vi "SVFA Concatenate Spectra (XY) (1 Ch).vi"(10 "spectrum (high frequency)":cluster{"X":dbl[], "Y":dbl[]}, 11 "spectrum (low frequency)":cluster{"X":dbl[], "Y":dbl[]}) -> (3 "concatenated spectrum":cluster{"X":dbl[], "Y":dbl[]})   [LabVIEW 2017]
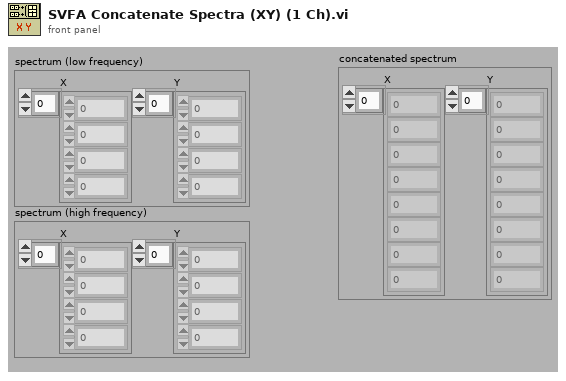
[diagram p1: front panel]
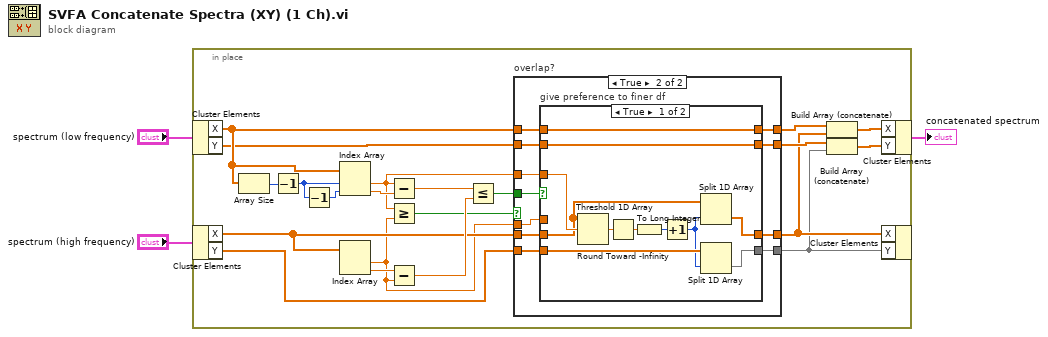
[diagram p0: block diagram]
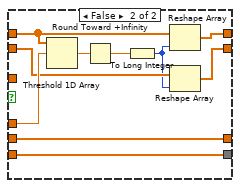
[diagram p3: hidden frame]
diagram:
  n1 = in-place {
    n2 = in-place-cluster #1("spectrum (low frequency)") -> ("X"=w14:dbl[], "Y"=w12:dbl[])
    n3 = in-place-cluster #2("spectrum (high frequency)") -> ("X"=w10:dbl[], "Y"=w7:dbl[])
    n4 = Array Size(array=w14) -> (size(s)=w22:i32)
    n5 = Decrement(x=w22) -> (x-1=w21:i32)
    n6 = Decrement(x=w21) -> (x-1=w20:i32)
    n7 = Index Array(array=w14, index #1=w21, index #2=w20) -> (element #1=w6:dbl, element #2=w18:dbl)
    n8 = Index Array(array=w10) -> (element #1=w5:dbl, element #2=w19:dbl)  [unwired: 2 in]
    n9 = Subtract(x=w6, y=w18) -> (x-y=w17:dbl)
    n10 = Greater Or Equal?(x=w6, y=w5) -> (x >= y?=w4:bool)
    n11 = Subtract(x=w19, y=w5) -> (x-y=w16:dbl)
    n12 = Less Or Equal?(x=w17, y=w16) -> (x <= y?=w15:bool)
    n13 = case "overlap?" shown="True" w4 {
      tunnel: w15 -> [_ w39]
      tunnel: w14 -> [w28 w38]
      tunnel: [w28 w37] -> w13
      tunnel: w12 -> [w27 w36]
      tunnel: [w27 w35] -> w11
      tunnel: w10 -> [w26 w34]
      tunnel: [w26 w33] -> w9
      tunnel: [w25 w32] -> w8
      tunnel: w7 -> [w25 w31]
      tunnel: w6 -> [_ w30]
      tunnel: w5 -> [_ w29]
      frame False {
      }
      frame True {
        n14 = case "give preference to finer df" shown="True" w39 {
          tunnel: w34 -> [w49 w55]
          tunnel: w30 -> [w50 _]
          tunnel: [w48 w55] -> w33
          tunnel: w31 -> [w44 w54]
          tunnel: [w47 w54] -> w32
          tunnel: w29 -> [_ w58]
          tunnel: w38 -> [w46 w57]
          tunnel: [w46 w53] -> w37
          tunnel: w36 -> [w45 w56]
          tunnel: [w45 w52] -> w35
          frame True {
            n15 = Threshold 1D Array(2:w50, 3:w49) -> (0:w43:dbl)  [unwired: 1 in]
            n16 = Round Toward -Infinity(1:w43) -> (0:w42:dbl)
            n17 = To Long Integer(number=w42) -> (32bit integer=w41:i32)
            n18 = Increment(x=w41) -> (x+1=w40:i32)
            n19 = Split 1D Array(array=w49, index=w40) -> (second subarray=w48:dbl[])  [unwired: 1 out]
            n20 = Split 1D Array(array=w44, index=w40) -> (second subarray=w47:dbl[])  [unwired: 1 out]
          }
          frame False {
            n21 = Threshold 1D Array(2:w58, 3:w57) -> (0:w60:dbl)  [unwired: 1 in]
            n22 = Round Toward +Infinity(x=w60) -> (ceil(x): smallest int >= x=w59:dbl)
            n23 = To Long Integer(number=w59) -> (32bit integer=w51:i32)
            n24 = Reshape Array(w57, w51) -> (w53:dbl[])
            n25 = Reshape Array(w56, w51) -> (w52:dbl[])
          }
        }
      }
    }
    n26 = Build Array (concatenate)(w13, w9) -> (w24:dbl[])
    n27 = Build Array (concatenate)(w11, w8) -> (w23:dbl[])
    n28 = in-place-cluster #1("X"=w24, "Y"=w23) -> (→"concatenated spectrum":cluster{"X":dbl[], "Y":dbl[]})
    n29 = in-place-cluster #2("X"=w9, "Y"=w8) -> ()  [unwired: 1 out]
  }
